vi "Local MS Operation.vi"(6 "PID Cluster":T3={"L1 to L4 PID Cluster"={"L1 PID Gains"={"Kp"=0.005, "Kd"=0.5, "Ki"=0.0005}, "L2 PID Gains"={"Kp"=0.01, "Kd"=1.0, "Ki"=0.005}, "L3 PID Gains"={"Kp"=0.05, "Kd"=1.0, "Ki"=0.0005}, "L4 PID Gains"={"Kp"=0.1, "Kd"=0.1, "Ki"=0.0005}}, "Stage PID Cluster"={"Stage Z PID"={"Kp"=0.0005, "Kd"=0.001, "Ki"=0.0}, "Stage Y PID"={"Kp"=0.0003, "Kd"=0.01, "Ki"=0.0}, "Stage X PID"={"Kp"=0.0003, "Kd"=0.01, "Ki"=0.0}}, "OCT Z PID Gains"={"Kp"=0.0003, "Kd"=0.0001, "Ki"=0.01}}, 8 "error in":errorcluster, 9 "Offset Home 2 RCM":dbl[](array[numeric])=[0.0, 0.0, 0.0, 0.0], 10 "Prev Posit Cluster":T2={"Prev L1 to L4 Posit"=[-0.5319, -0.035669172703475985, -2.0566170657346783, 0.9099264705882353], "Prev Stage Posit"=[6.002553885707208, 5.996566124542428, 5.995469940427586], "Prev OCT Z Posit"=-0.0}, 11 "FPGA VI Reference In":refnum<k20>) -> (0 "error out":errorcluster, 2 "Last Posit Cluster":T1={"Last L1 to L4 Posit"=[0.0, 0.0, 0.0, 0.0], "Last Stage Posit"=[6.0, 6.0, 6.0], "Last OCT Z Posit"=0.0}, 3 "FPGA VI Reference Out":refnum<k20>)   [LabVIEW 2016]
uses:
  <vilib>/Platform/TimedLoop/XDataNode/timing_clust.ctl
  <vilib>/Platform/TimedLoop/XDataNode/nitl_modes.ctl
  <vilib>/Platform/TimedLoop/XDataNode/wakeup.ctl
  Global Variables.vi
  <vilib>/Utility/error.llb/Error Cluster From Error Code.vi
  <vilib>/rvi/errors/niLvFpgaAdjustHostInterfaceError.vi
  <vilib>/platform/TimedLoop/XDataNode/XDataNode.xnode
  <vilib>/rvi/interface/nirviReadWriteControl/nirviReadWriteControl.xnode
  FPGA Bitfiles/PhantomControlPI_FPGATarget_QuadCtr2_E2412E44.lvbitx
  IRISS_FPGA_IO.vi
  <vilib>/Platform/TimedLoop/XDataNode/XDNodeRunTimeDep.lvlib
  Library/KevinLibraryAll/labview/KevLib01.lvlib
  NiFpgaLv.dll
panel:
  out "Period [ms]":i64=10
  out "L1 to L4 Remote cmd":dbl[](array[numeric])
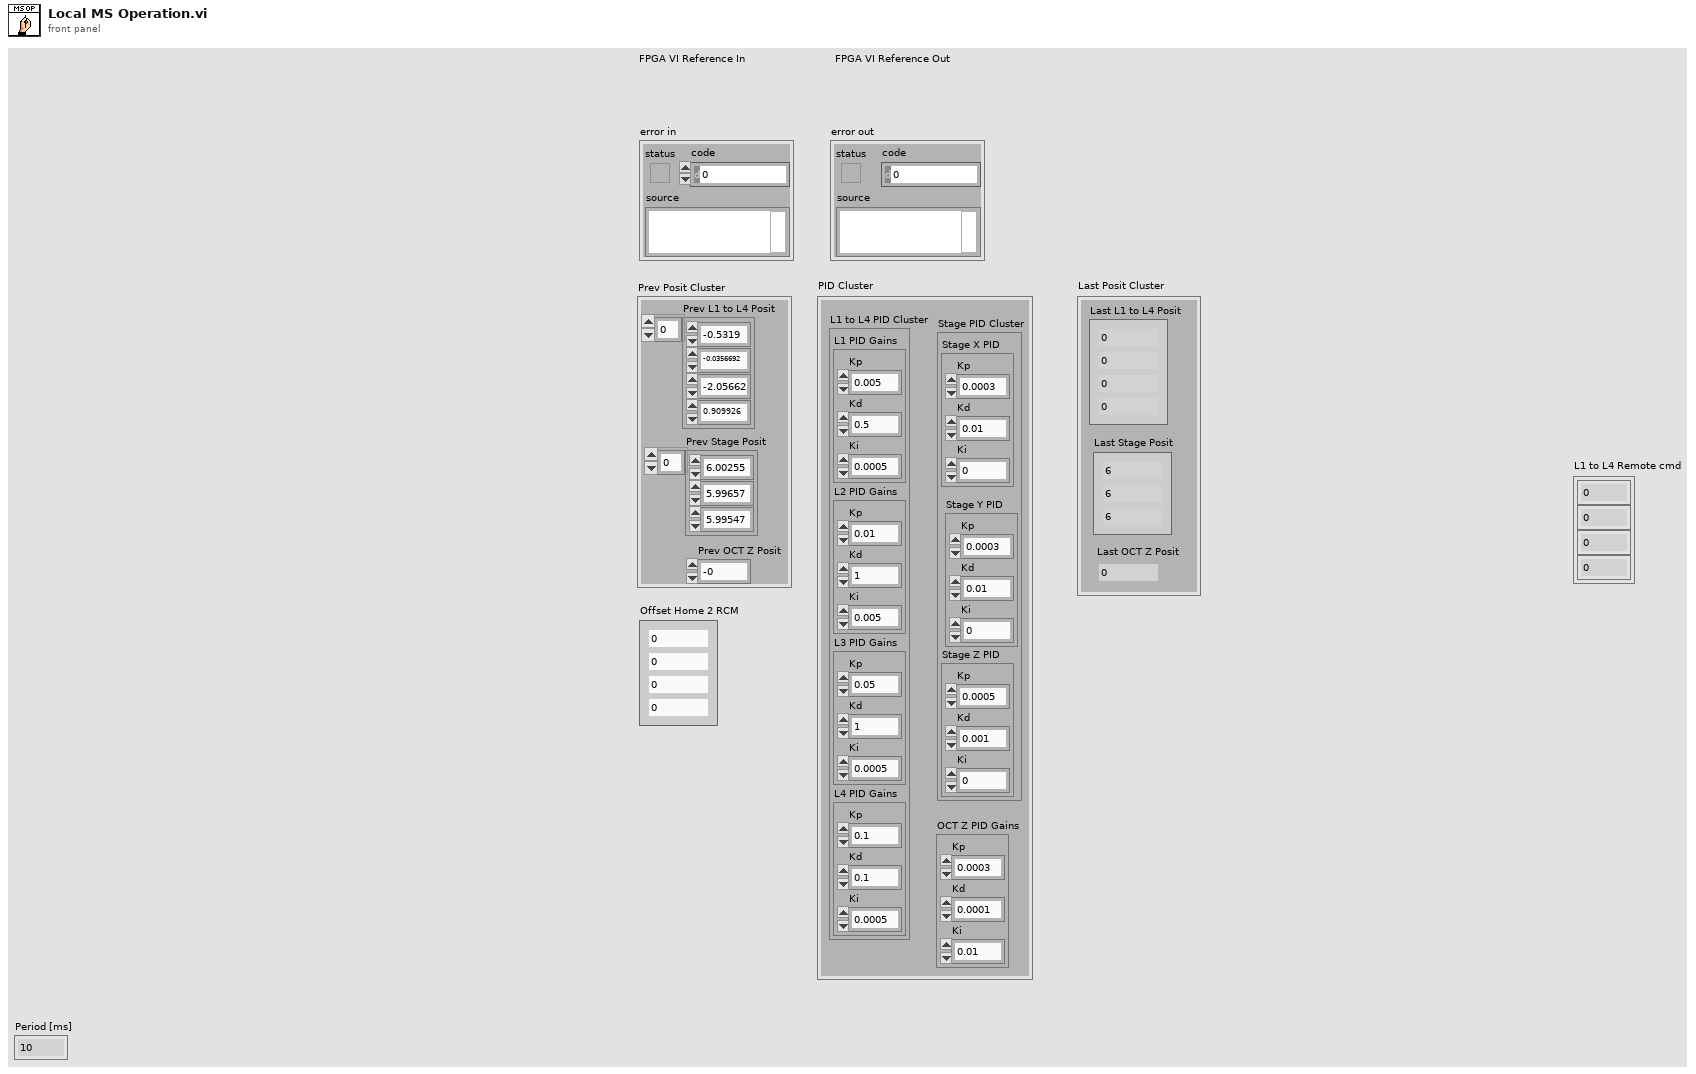
[diagram p1: front panel]
types:
  T1 = cluster{"Last L1 to L4 Posit":dbl[], "Last Stage Posit":dbl[], "Last OCT Z Posit":dbl}
  T2 = cluster{"Prev L1 to L4 Posit":dbl[], "Prev Stage Posit":dbl[], "Prev OCT Z Posit":dbl}
  T3 = cluster{"L1 to L4 PID Cluster":cluster{"L1 PID Gains":cluster{"Kp":dbl, "Kd":dbl, "Ki":dbl}, "L2 PID Gains":cluster{"Kp":dbl, "Kd":dbl, "Ki":dbl}, "L3 PID Gains":cluster{"Kp":dbl, "Kd":dbl, "Ki":dbl}, "L4 PID Gains":cluster{"Kp":dbl, "Kd":dbl, "Ki":dbl}}, "Stage PID Cluster":cluster{"Stage Z PID":cluster{"Kp":dbl, "Kd":dbl, "Ki":dbl}, "Stage Y PID":cluster{"Kp":dbl, "Kd":dbl, "Ki":dbl}, "Stage X PID":cluster{"Kp":dbl, "Kd":dbl, "Ki":dbl}}, "OCT Z PID Gains":cluster{"Kp":dbl, "Kd":dbl, "Ki":dbl}}
  T4 = typedef "XDNodeRunTimeDep.lvlib/timing_clust.ctl" = cluster{"Expected End [f-1]":u64, "Actual End [f-1]":u64, "Finished Late? [f-1]":bool, "Expected End [i-1]":u64, "Actual End [i-1]":u64, "Finished Late? [i-1]":bool, "Expected Start [i]":u64, "Actual Start [i]":u64, "Expected Start [f]":u64, "Actual Start [f]":u64, "Source Name":string, "Structure Name":string, "Period":i64, "Deadline":i64, "Offset":i64, "Start":i64, "Priority":i32, "Timeout":i32, "Mode":T5, "Wakeup Reason":T6, "Error":errorcluster, "Source Type":string, "Secondary Source Type":string, "Global End Time":u64, "Global Start Time":u64, "Frame Duration":u64, "Iteration Duration":u64, "Assigned CPU":i32, "I/O Scan Engine Mode":u32}
  T5 = typedef "XDNodeRunTimeDep.lvlib/nitl_modes.ctl" = enum32{"No Change", "Process missed periods, maintain original phase", "Discard missed periods, maintain original phase", "Process missed periods, ignore original phase", "Discard missed periods, ignore original phase"}
  T6 = typedef "XDNodeRunTimeDep.lvlib/wakeup.ctl" = enum32{"Normal", "Aborted", "Asynchronous wakeup", "Timing source error", "Timed loop error", "Timeout"}
  T7 = cluster{"L1 PID Gains":cluster{"Kp":dbl, "Kd":dbl, "Ki":dbl}, "L2 PID Gains":cluster{"Kp":dbl, "Kd":dbl, "Ki":dbl}, "L3 PID Gains":cluster{"Kp":dbl, "Kd":dbl, "Ki":dbl}, "L4 PID Gains":cluster{"Kp":dbl, "Kd":dbl, "Ki":dbl}}
  T8 = cluster{"Stage Z PID":cluster{"Kp":dbl, "Kd":dbl, "Ki":dbl}, "Stage Y PID":cluster{"Kp":dbl, "Kd":dbl, "Ki":dbl}, "Stage X PID":cluster{"Kp":dbl, "Kd":dbl, "Ki":dbl}}
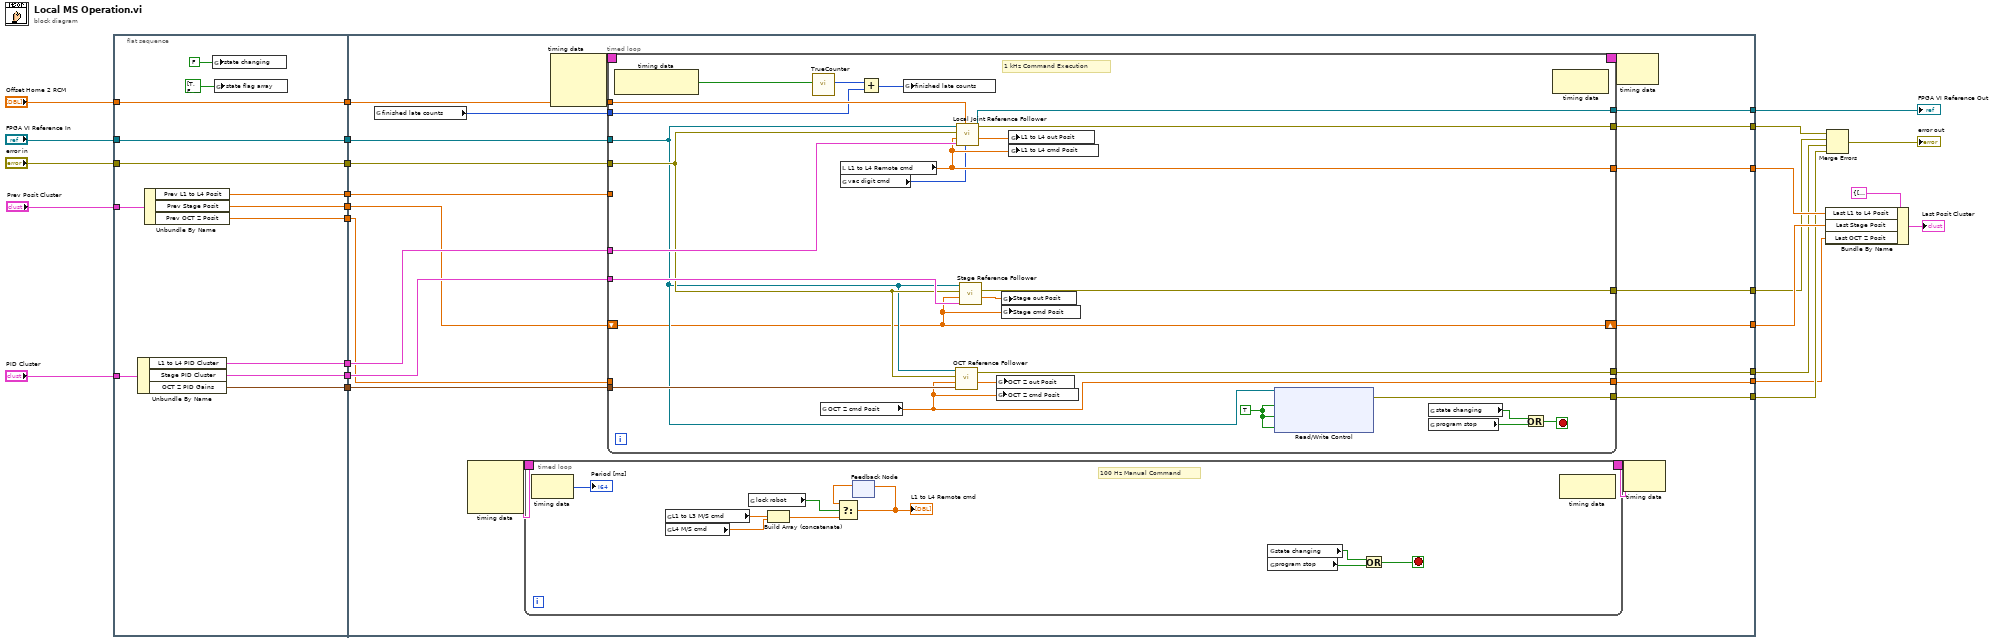
[diagram p0: block diagram]
diagram:
  n1 = flat-sequence {
    tunnel: [w36] -> w25
    tunnel: "FPGA VI Reference In" -> [w36]
    tunnel: [w35] -> w23
    tunnel: "error in" -> [w35]
    tunnel: [w31] -> w21
    tunnel: "Offset Home 2 RCM" -> [w31]
    tunnel: "Prev Posit Cluster" -> [w28]
    tunnel: [w34] -> w18
    tunnel: "PID Cluster" -> [w33]
    tunnel: [w32] -> w16
    tunnel: [w30] -> w4
    tunnel: [w29] -> w3
    tunnel: [w27] -> w2
    tunnel: [w26] -> w1
    tunnel: w25 -> [w40]
    tunnel: w23 -> [w39]
    tunnel: w21 -> [w56]
    tunnel: w18 -> [w55]
    tunnel: w16 -> [w54]
    tunnel: [w53] -> w6
    tunnel: [w52] -> w12
    tunnel: [w51] -> w13
    tunnel: [w41] -> w10
    tunnel: [w42] -> w9
    tunnel: [w50] -> w7
    tunnel: [w49] -> w8
    tunnel: [w43] -> w5
    tunnel: w4 -> [w48]
    tunnel: w3 -> [w47]
    tunnel: w2 -> [w45]
    tunnel: w1 -> [w44]
    frame #0 {
      n2 = Unbundle By Name(w33) -> ("L1 to L4 PID Cluster"=w32:T7, "Stage PID Cluster"=w30:T8, "OCT Z PID Gains"=w29:cluster{"Kp":dbl, "Kd":dbl, "Ki":dbl})
      n3 = Unbundle By Name(w28) -> ("Prev L1 to L4 Posit"=w34:dbl[], "Prev Stage Posit"=w27:dbl[], "Prev OCT Z Posit"=w26:dbl)
      n4 = global write "Global Variables.vi" "state changing"(FALSE ("state changing")) -> ()
      n5 = global write "Global Variables.vi" "state flag array"(bool[] [TRUE, FALSE, FALSE, FALSE, FALSE, FALSE, FALSE, FALSE, FALSE] ("state flag array")) -> ()
    }
    frame #1 {
      n6 = global read "Global Variables.vi" "finished late counts"() -> (w46:u16)
      n7 = node-c288() -> (w58:T4)  [unwired: 3 in]
      n8 = timed-loop {
        timing: w58 -> [_]
        timing-out: [_] -> w57
        stop <- w70 stop-if-true
        # "100 Hz Manual Command"
        n9 = node-c288() -> (→"Period [ms]":i64)  [unwired: 1 in]
        n10 = global read "Global Variables.vi" "L1 to L3 M/S cmd"() -> (w63:dbl[])
        n11 = global read "Global Variables.vi" "L4 M/S cmd"() -> (w62:dbl)
        n12 = global read "Global Variables.vi" "lock robot"() -> (w61:bool)
        n13 = Build Array (concatenate)(w63, w62) -> (w66:dbl[])
        n14 = feedback #1() -> (w68:dbl[])  [unwired: 1 in]
        n15 = Select(t=w68, s=w61, f=w66) -> (s? t:f=w67:dbl[])
        "L1 to L4 Remote cmd" <- w67
        n16 = feedback-in #1(w67) -> ()
        n17 = global read "Global Variables.vi" "state changing"() -> (w69:bool)
        n18 = global read "Global Variables.vi" "program stop"() -> (w65:bool)
        n19 = Or(x=w69, y=w65) -> (x .or. y?=w70:bool)
        n20 = node-c288() -> ()  [unwired: 1 in, 1 out]
      }
      n21 = node-c288() -> (w60:T4)  [unwired: 3 in]
      n22 = timed-loop {
        timing: w60 -> [_]
        timing-out: [_] -> w59
        tunnel: w40 -> [w84]
        tunnel: w39 -> [w85]
        tunnel: w56 -> [w99]
        tunnel: w55 -> [_]
        tunnel: w54 -> [w98]
        tunnel: [w97] -> w53
        tunnel: [w96] -> w52
        tunnel: [w95] -> w51
        tunnel: [w94] -> w50
        tunnel: [w93] -> w49
        tunnel: w48 -> [w91]
        tunnel: w47 -> [w90]
        tunnel: w46 -> [w86]
        shift-right: [w79] -> w42
        shift-left: w45 -> [w79]
        tunnel: [w80] -> w41
        tunnel: w44 -> [_]
        tunnel: [w76] -> w43
        stop <- w101 stop-if-true
        w78 = TRUE ("Conn0/DIO15 Button 4")
        # "1 kHz Command Execution"
        n23 = node-c288() -> (w89:bool)  [unwired: 1 in]
        n24 = call "TrueCounter.vi"("True?"=w89) -> ("True Count"=w87:u16)  [unwired: 10 in]
        n25 = global read "Global Variables.vi" "OCT Z cmd Posit"() -> (w76:dbl)
        n26 = local read "L1 to L4 Remote cmd"() -> (w80:dbl[])
        n27 = global read "Global Variables.vi" "vac digit cmd"() -> (w77:i8)
        n28 = Add(x=w87, y=w86) -> (x+y=w88:u16)
        n29 = global write "Global Variables.vi" "finished late counts"(w88) -> ()
        n30 = call "OCT Reference Follower.vi"("OCT Z PID Gains"=w90, "OCT  Z cmd Posit [mm]"=w76, "error in"=w85, "FPGA VI Reference In"=w84) -> ("OCT  Z out Posit [mm]"=w83:dbl, "error out"=w94:errorcluster)  [unwired: 5 in, 1 out]
        n31 = call "Local Joint Reference Follower.vi"("Digital Cmd [0-78]"=w77, "Offset Home2RCM [deg/mm]"=w99, "PID Ctrl Cluster"=w98, "Ref Array [deg/mm]"=w80, "error in"=w85, "FPGA VI Reference In"=w84) -> ("Output Posit Array [deg/mm]"=w81:dbl[], "error out"=w96:errorcluster, "FPGA VI Reference Out"=w95:refnum<k20>)  [unwired: 3 in]
        n32 = call "Stage Reference Follower.vi"("Stage PID Cluster"=w91, "Stage cmd Posit [mm]"=w79, "error in"=w85, "FPGA VI Reference In"=w84) -> ("Stage out Posit [mm]"=w82:dbl[], "error out"=w93:errorcluster)  [unwired: 5 in, 1 out]
        n33 = global write "Global Variables.vi" "OCT Z cmd Posit"(w76) -> ()
        n34 = global write "Global Variables.vi" "OCT Z out Posit"(w83) -> ()
        n35 = global write "Global Variables.vi" "Stage out Posit"(w82) -> ()
        n36 = global write "Global Variables.vi" "Stage cmd Posit"(w79) -> ()
        n37 = global write "Global Variables.vi" "L1 to L4 out Posit"(w81) -> ()
        n38 = global write "Global Variables.vi" "L1 to L4 cmd Posit"(w80) -> ()
        n39 = xnode "Read/Write Control"("FPGA VI Reference In"=w84, "Conn0/DIO12 Button 1"=w78, "Conn0/DIO13 Button 2"=w78, "Conn0/DIO15 Button 4"=w78) -> ("error out"=w97:errorcluster)  [unwired: 1 in, 1 out]
        n40 = global read "Global Variables.vi" "state changing"() -> (w100:bool)
        n41 = global read "Global Variables.vi" "program stop"() -> (w92:bool)
        n42 = Or(x=w100, y=w92) -> (x .or. y?=w101:bool)
        n43 = node-c288() -> ()  [unwired: 1 in, 1 out]
      }
      n44 = node-c288(w59) -> ()  [unwired: 1 out]
      n45 = node-c288(w57) -> ()  [unwired: 1 out]
    }
  }
  n46 = Bundle By Name(cluster=T1 {"Last L1 to L4 Posit"=[-0.5607, -0.038216970753724266, -2.0806193533568895, 1.1787683823529411], "Last Stage Posit"=[6.002553885707208, 5.996566124542428, 5.995469940427586], "Last OCT Z Posit"=-0.0} ("Last Posit Cluster 2"), "Last L1 to L4 Posit"=w10, "Last Stage Posit"=w9, "Last OCT Z Posit"=w5) -> (→"Last Posit Cluster":T1)
  n47 = Merge Errors(w12, w8, w7, w6) -> (→"error out":errorcluster)
  "FPGA VI Reference Out" <- w13
